vi "Set Column Property.vi"(8 "error in":errorcluster, 9 "Value":variant, 10 "Property":string, 11 "Sourcegrid in":refnum<class "Sourcegrid.lvclass">) -> (0 "error out":errorcluster, 3 "Sourcegrid out":refnum<class "Sourcegrid.lvclass">)   [LabVIEW 2024, in "Sourcegrid.lvclass"]
uses:
  Sourcegrid.lvclass
  Sourcegrid.lvclass/Sourcegrid.ctl
  D:/git/Sourcegrid-LabVIEW/dll/SourceGrid.dll
  dll/SourceGrid.dll
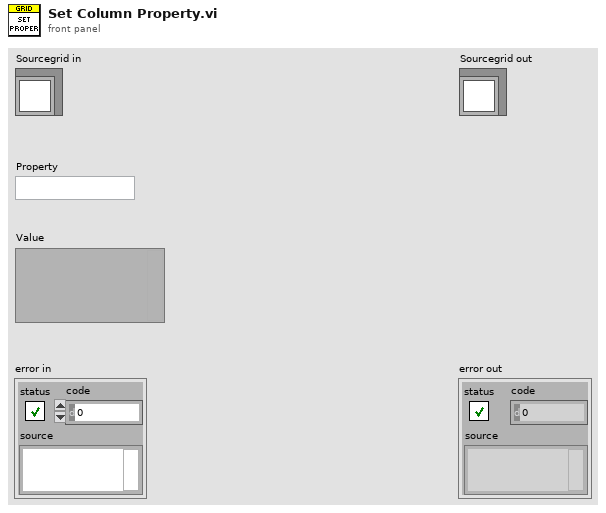
[diagram p1: front panel]
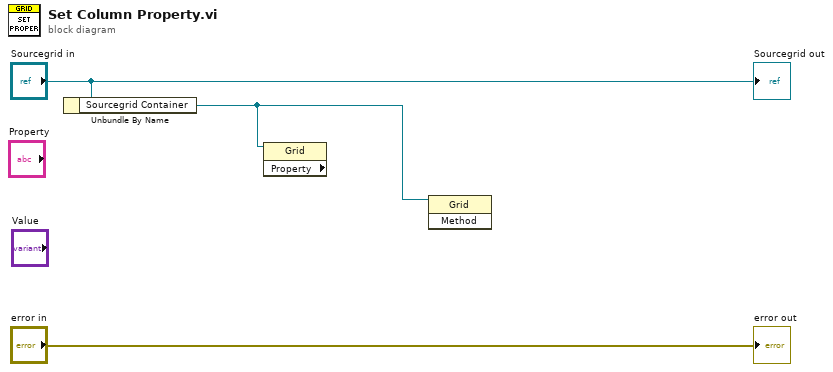
[diagram p0: block diagram]
diagram:
  n1 = Unbundle By Name("Sourcegrid in") -> ("Sourcegrid Container"=w1:refnum<k24>)
  n2 = property class="Grid" props=[](reference=w1) -> ()  [unwired: 1 in, 3 out]
  n3 = invoke class="Grid" method=#-1(reference=w1) -> ()  [unwired: 2 in, 3 out]
  "error out" <- "error in"
  "Sourcegrid out" <- "Sourcegrid in"
